vi "Define Config.vi"(8 "ErrorIn":errorcluster, 9 "Config":refnum<class "IConfig.lvclass">, 10 "Name":string, 11 "TopModuleIn":refnum<class "TopModule.lvclass">) -> (0 "ErrorOut":errorcluster, 3 "TopModuleOut":refnum<class "TopModule.lvclass">)   [LabVIEW 2019, in "TopModule.lvclass"]
uses:
  TopModule.lvclass
  IConfig/IConfig.lvclass
  TopModule.lvclass/TopModule.ctl
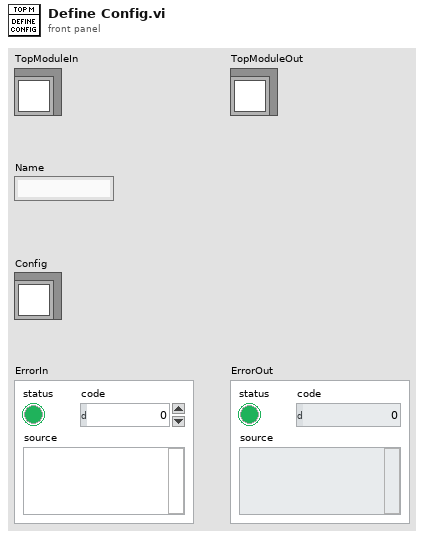
[diagram p1: front panel]
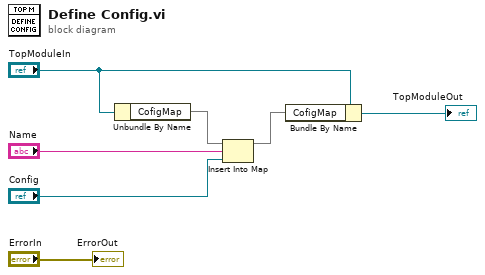
[diagram p0: block diagram]
diagram:
  n1 = Unbundle By Name("TopModuleIn") -> ("CofigMap"=w5:map{string, refnum<class "IConfig.lvclass">})
  n2 = Insert Into Map(map in=w5, key="Name", value="Config") -> (map out=w6:map{string, refnum<class "IConfig.lvclass">})  [unwired: 2 out]
  n3 = Bundle By Name(cluster="TopModuleIn", "CofigMap"=w6) -> (→"TopModuleOut":refnum<class "TopModule.lvclass">)
  "ErrorOut" <- "ErrorIn"
